vi "Listbox.Set.vi"(5 "Force?":bool, 7 "UI.Listbox":refnum<vi>, 8 "error in (no error)":errorcluster, 9 "List":T2, 10 "Value":i64, 11 "WorkspaceManager":T1) -> (0 "error out":errorcluster, 3 "WorkspaceManager out":T1)   [LabVIEW 2015, in "Workspace.Obejct.Radio.lvlib"]
uses:
  Workspace.Obejct.Radio.lvlib
  Types/Config.ctl
  <vilib>/NI Veristand/Execution/Workspace/WorkspaceAPI.ctl
  NationalInstruments.VeriStand.ClientAPI
  <vilib>/NI Veristand/Execution/Workspace/NI_VS Workspace ExecutionAPI.lvlib
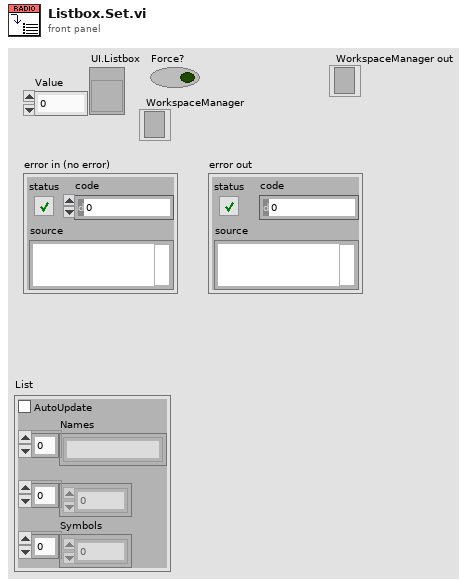
[diagram p1: front panel]
types:
  T1 = typedef "NI_VS Workspace ExecutionAPI.lvlib/WorkspaceAPI.ctl" = refnum<k24>
  T2 = typedef "Workspace.Obejct.Radio.lvlib/Config.ctl" = cluster{"AutoUpdate":bool, "Names":string[], "Values":dbl[], "Symbols":i32[]}
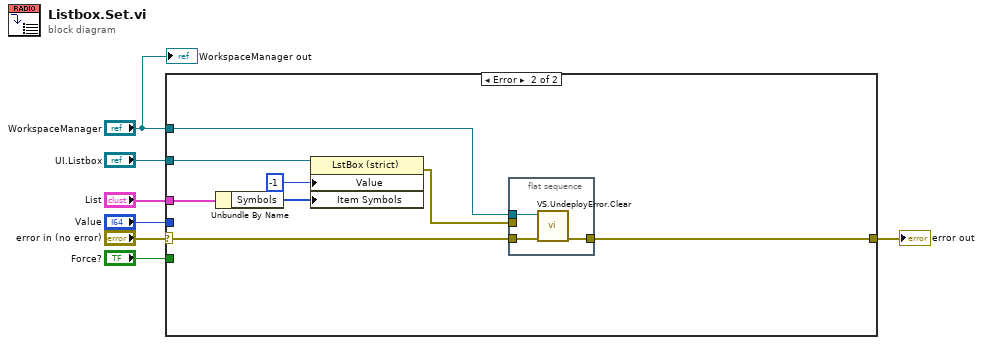
[diagram p0: block diagram]
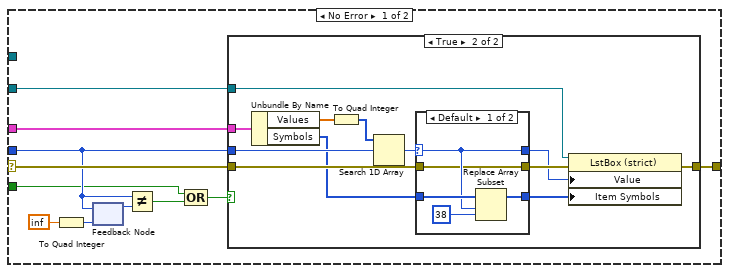
[diagram p2: hidden frame]
diagram:
  n1 = case shown="Error" "error in (no error)" {
    selector: "error in (no error)" -> [w15 w44]
    tunnel: "Value" -> [w13 _]
    tunnel: [w12 w45] -> w2
    tunnel: "List" -> [w14 w47]
    tunnel: "Force?" -> [w9 _]
    tunnel: "WorkspaceManager" -> [_ w46]
    tunnel: "UI.Listbox" -> [w8 w41]
    frame No Error {
      n2 = To Quad Integer(1:inf) -> (0:w16:i64)
      n3 = feedback #1(w16) -> (w17:i64)
      n4 = feedback-in #1(w13) -> ()
      n5 = Not Equal?(x=w13, y=w17) -> (x != y?=w11:bool)
      n6 = Compound Arithmetic op=OR(w9, w11) -> (w10:bool)
      n7 = case shown="True" w10 {
        tunnel: w15 -> [w19 w26]
        tunnel: w14 -> [_ w31]
        tunnel: w13 -> [_ w28]
        tunnel: [w19 w23] -> w12
        tunnel: w8 -> [_ w20]
        frame False {
        }
        frame True {
          n8 = Unbundle By Name(w31) -> ("Values"=w30:dbl[], "Symbols"=w25:i32[])
          n9 = To Quad Integer(1:w30) -> (0:w29:i64[])
          n10 = Search 1D Array(1D array=w29, element=w28) -> (index of element=w27:i32)  [unwired: 1 in]
          n11 = case shown="Default" w27 {
            selector: w27 -> [w33 w38]
            tunnel: w25 -> [w36 w39]
            tunnel: [w35 w39] -> w21
            tunnel: [w33 w38] -> w22
            tunnel: [w32 w37] -> w24
            tunnel: w26 -> [w32 w37]
            frame Default {
              n12 = Replace Array Subset(array=w36, new element=38 ("new element/subarray"), index=w33) -> (w35:i32[])
            }
            frame -1 {
            }
          }
          n13 = property class="LstBox (strict)"(reference=w20, error in=w24, "Value"=w22, "Item Symbols"=w21) -> (error out=w23:errorcluster)  [unwired: 1 out]
        }
      }
    }
    frame Error {
      n14 = Unbundle By Name(w47) -> ("Symbols"=w43:i32[])
      n15 = property class="LstBox (strict)"(reference=w41, "Value"=-1 ("index of element"), "Item Symbols"=w43) -> (error out=w40:errorcluster)  [unwired: 1 in, 1 out]
      n16 = flat-sequence {
        tunnel: w46 -> [w50]
        tunnel: [w49] -> w45
        tunnel: w44 -> [w48]
        tunnel: w40 -> [_]
        frame #0 {
          n17 = call "VS.UndeployError.Clear.vi"("error in (no error)"=w48, "WorkspaceManager in"=w50) -> ("error out"=w49:errorcluster)  [unwired: 8 in, 1 out]
        }
      }
    }
  }
  "error out" <- w2
  "WorkspaceManager out" <- "WorkspaceManager"
